vi "Control Labels.vi"(11 "myRIOMetaDataObj.lvclass":refnum<class "myRIOMetaDataObj.lvclass">) -> (2 "localized control labels":string[](array[string]), 3 "DNL_unlocalized control labels":string[](array[string]), 4 "DNL_unlocalized string constant labels":string[](array[string]), 6 "localized string constant values":string[](array[string]))   [LabVIEW 2021, in "myRIOMetaDataObj.lvclass"]
doc: "Override this VI to supply the control label localizations. The first array is the label text as it appears in your unmodified template VIs. The second array is the label text as it should appear in the user's instantiated VIs. You may dynamically generate the second array based on user values obtained through the New Project Wizard and your spec page VI."
uses:
  myRIOMetaDataObj.lvclass
  <resource>/dialog/NewProjectWizard/MetaDataObj/MetaDataObj.lvclass
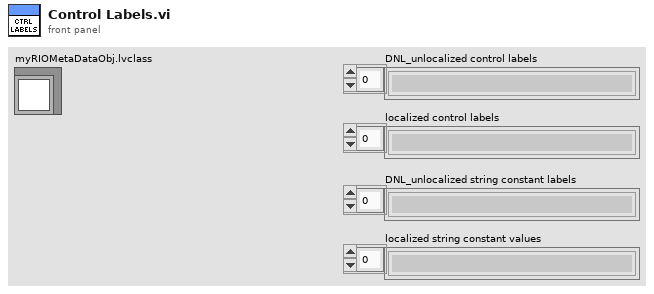
[diagram p1: front panel]
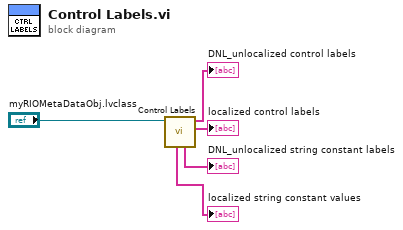
[diagram p0: block diagram]
diagram:
  n1 = call-parent "Control Labels.vi"("MetaDataObj.lvclass"="myRIOMetaDataObj.lvclass") -> ("localized control labels"=→"localized control labels":string[], "DNL_unlocalized control labels"=→"DNL_unlocalized control labels":string[], "DNL_unlocalized string constant labels"=→"DNL_unlocalized string constant labels":string[], "localized string constant values"=→"localized string constant values":string[])  [unwired: 7 in]
